vi "SaveHands_modified.vi"(8 "Error In":errorcluster, 11 ".NET Refnum in":refnum<k24>) -> (0 "Error Out":errorcluster, 3 "Left Hand":T1={"Palm Normal"={"Pitch"=nan, "Yaw"=nan, "Roll"=nan, "Magnitude"=nan, "XYZ"=[nan, nan, nan]}, "Palm Position"={"Pitch"=nan, "Yaw"=nan, "Roll"=nan, "Magnitude"=nan, "XYZ"=[nan, nan, nan]}, "Palm Velocity"={"Pitch"=nan, "Yaw"=nan, "Roll"=nan, "Magnitude"=nan, "XYZ"=[nan, nan, nan]}, "Direction"={"Pitch"=nan, "Yaw"=nan, "Roll"=nan, "Magnitude"=nan, "XYZ"=[nan, nan, nan]}, "Palm Position (Stabilized)"={"Pitch"=nan, "Yaw"=nan, "Roll"=nan, "Magnitude"=nan, "XYZ"=[nan, nan, nan]}, "Sphere Center"={"Pitch"=nan, "Yaw"=nan, "Roll"=nan, "Magnitude"=nan, "XYZ"=[nan, nan, nan]}, "Pointables"=[], "ID"=0, "Time Visible"=0.0, "Sphere Radius"=0.0})   [LabVIEW 2015]
uses:
  <vilib>/MakerHub/Leap/Private/Type Defs/Hand.ctl
  <vilib>/MakerHub/Leap/Private/Type Defs/Vector.ctl
  <vilib>/MakerHub/Leap/Private/Type Defs/Pointable.ctl
  <vilib>/MakerHub/Leap/Private/Type Defs/Pointable Type.ctl
  <vilib>/MakerHub/Leap/Private/Type Defs/Pointable Zone.ctl
  C:/Program Files (x86)/National Instruments/LabVIEW 2015/vi.lib/MakerHub/Leap/Private/Libs/LeapCSharp.NET3.5.dll
  Program Files (x86)/National Instruments/LabVIEW 2015/vi.lib/MakerHub/Leap/Private/Libs/LeapCSharp.NET3.5.dll
  <vilib>/MakerHub/Leap/LMH-Leap.lvlib
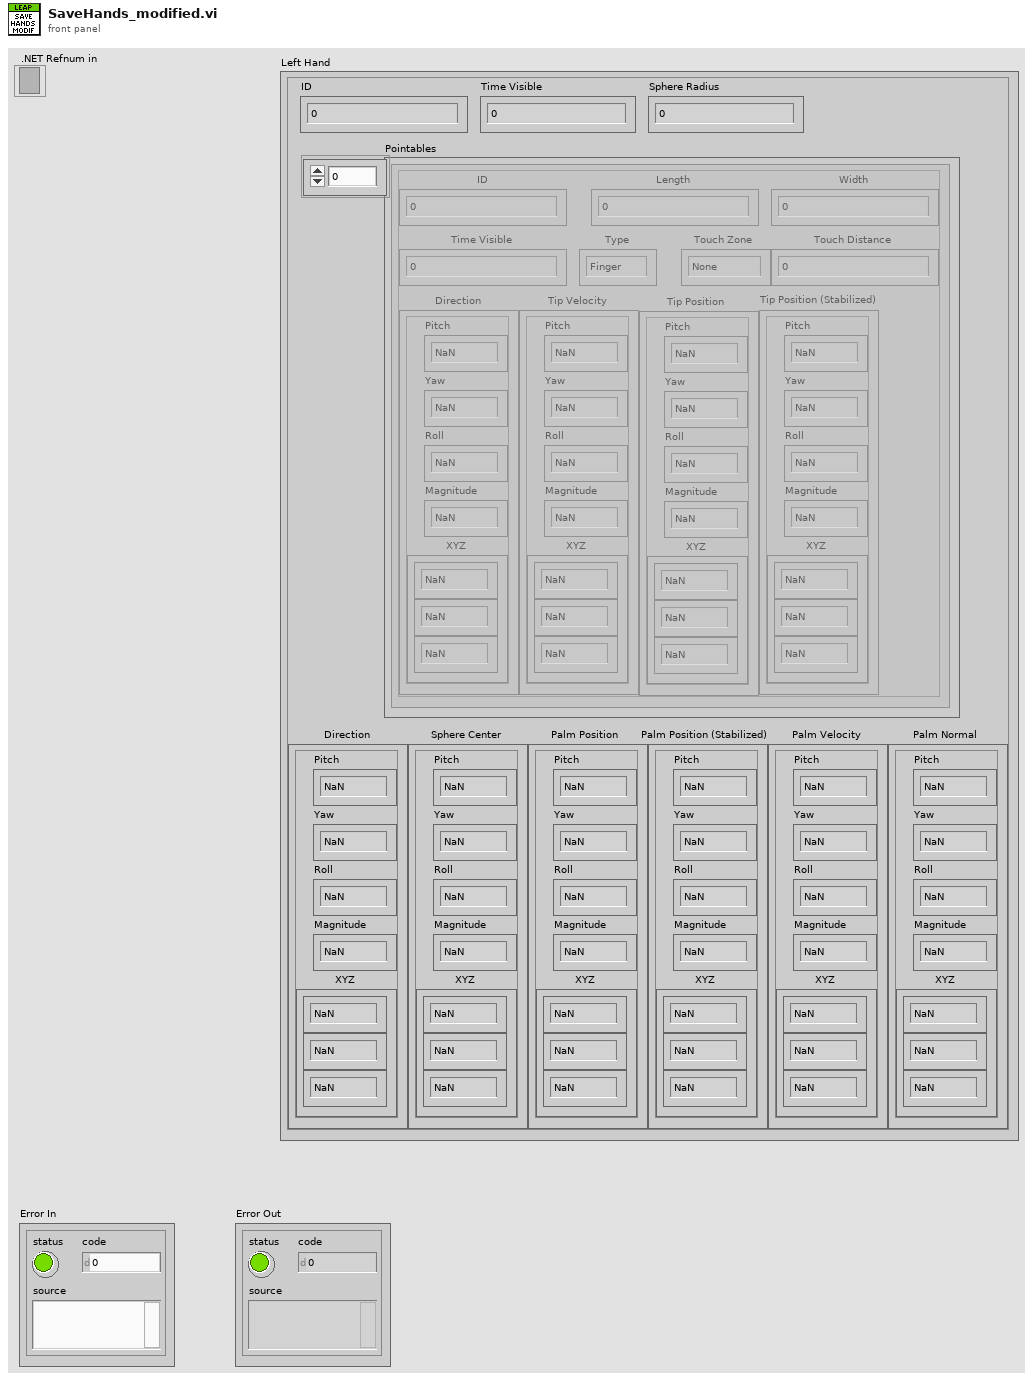
[diagram p1: front panel]
types:
  T1 = typedef "LMH-Leap.lvlib/Hand.ctl" = cluster{"Palm Normal":T2, "Palm Position":T2, "Palm Velocity":T2, "Direction":T2, "Palm Position (Stabilized)":T2, "Sphere Center":T2, "Pointables":T3[], "ID":i32, "Time Visible":sgl, "Sphere Radius":sgl}
  T2 = typedef "LMH-Leap.lvlib/Vector.ctl" = cluster{"Pitch":sgl, "Yaw":sgl, "Roll":sgl, "Magnitude":sgl, "XYZ":sgl[]}
  T3 = typedef "LMH-Leap.lvlib/Pointable.ctl" = cluster{"Type":T4, "Touch Zone":T5, "ID":i32, "Length":dbl, "Width":dbl, "Time Visible":dbl, "Touch Distance":dbl, "Direction":T2, "Tip Position":T2, "Tip Velocity":T2, "Tip Position (Stabilized)":T2}
  T4 = typedef "LMH-Leap.lvlib/Pointable Type.ctl" = enum16{"Finger", "Tool"}
  T5 = typedef "LMH-Leap.lvlib/Pointable Zone.ctl" = enum16{"None", "Hovering", "Touching"}
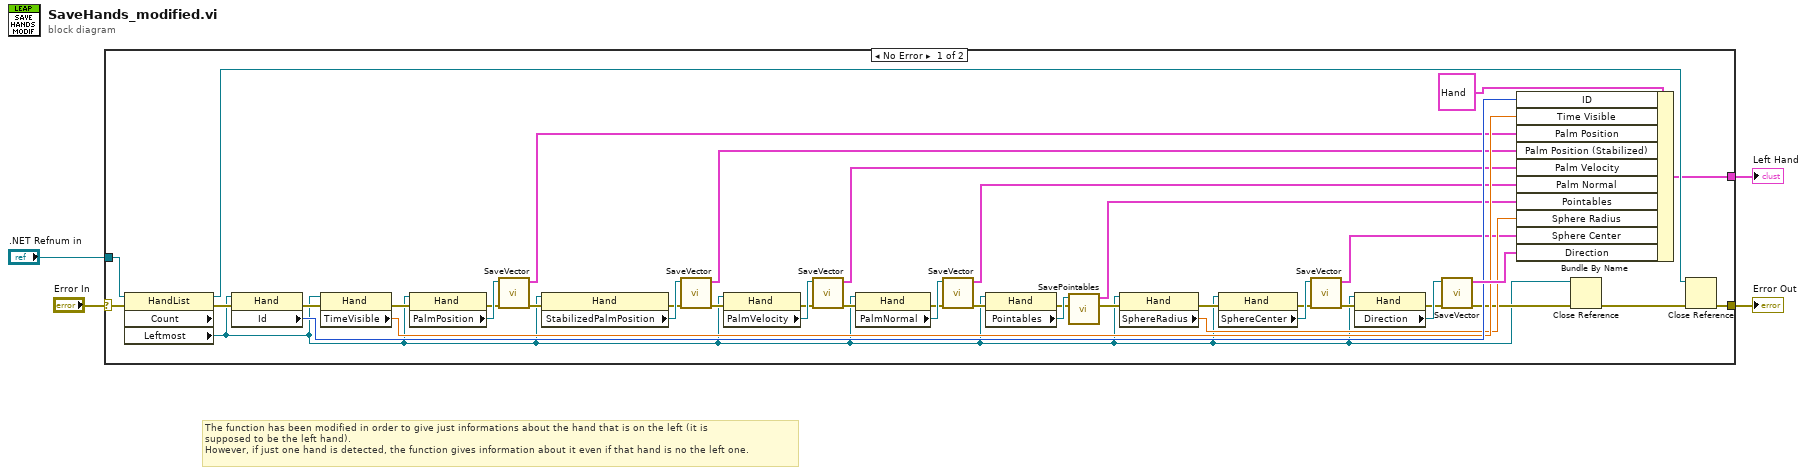
[diagram p0: block diagram]
diagram:
  # "The function has been modified in order to give just informations about the hand that is on the left (it is\nsupposed to be the left hand).\nHowever, if just one hand is detected, the function gives information about it even if that hand is no the left one."
  n1 = case shown="No Error" "Error In" {
    selector: "Error In" -> [w46 w48]
    tunnel: ".NET Refnum in" -> [w5 _]
    tunnel: [w44 w48] -> w3
    tunnel: [w8 _] -> w1
    frame No Error {
      n2 = property class="HandList" props=["Count", "Leftmost"](reference=w5, error in=w46) -> (reference out=w47:refnum<k24>, error out=w9:errorcluster, "Leftmost"=w6:refnum<k24>)  [unwired: 1 out]
      n3 = property class="Hand"(reference=w6, error in=w9) -> (error out=w41:errorcluster, "Id"=w38:i32)  [unwired: 1 out]
      n4 = property class="Hand"(reference=w6, error in=w41) -> (error out=w39:errorcluster, "TimeVisible"=w34:sgl)  [unwired: 1 out]
      n5 = property class="Hand"(reference=w6, error in=w39) -> (error out=w11:errorcluster, "PalmPosition"=w33:refnum<k24>)  [unwired: 1 out]
      n6 = call <vilib>:"SaveVector.vi"("error in (no error)"=w11, "Leap Vector"=w33) -> ("error out"=w10:errorcluster, "Vector"=w31:T2)  [unwired: 8 in]
      n7 = property class="Hand"(reference=w6, error in=w10) -> (error out=w12:errorcluster, "StabilizedPalmPosition"=w32:refnum<k24>)  [unwired: 1 out]
      n8 = call <vilib>:"SaveVector.vi"("error in (no error)"=w12, "Leap Vector"=w32) -> ("error out"=w13:errorcluster, "Vector"=w30:T2)  [unwired: 8 in]
      n9 = property class="Hand"(reference=w6, error in=w13) -> (error out=w14:errorcluster, "PalmVelocity"=w37:refnum<k24>)  [unwired: 1 out]
      n10 = call <vilib>:"SaveVector.vi"("error in (no error)"=w14, "Leap Vector"=w37) -> ("error out"=w15:errorcluster, "Vector"=w29:T2)  [unwired: 8 in]
      n11 = property class="Hand"(reference=w6, error in=w15) -> (error out=w16:errorcluster, "PalmNormal"=w36:refnum<k24>)  [unwired: 1 out]
      n12 = call <vilib>:"SaveVector.vi"("error in (no error)"=w16, "Leap Vector"=w36) -> ("error out"=w17:errorcluster, "Vector"=w28:T2)  [unwired: 8 in]
      n13 = property class="Hand"(reference=w6, error in=w17) -> (error out=w26:errorcluster, "Pointables"=w27:refnum<k24>)  [unwired: 1 out]
      n14 = call <vilib>:"SavePointables.vi"("error in (no error)"=w26, "Leap Pointables"=w27) -> ("error out"=w40:errorcluster, "Pointables"=w18:T3[])  [unwired: 8 in]
      n15 = property class="Hand"(reference=w6, error in=w40) -> (error out=w42:errorcluster, "SphereRadius"=w25:sgl)  [unwired: 1 out]
      n16 = property class="Hand"(reference=w6, error in=w42) -> (error out=w19:errorcluster, "SphereCenter"=w35:refnum<k24>)  [unwired: 1 out]
      n17 = call <vilib>:"SaveVector.vi"("error in (no error)"=w19, "Leap Vector"=w35) -> ("error out"=w20:errorcluster, "Vector"=w24:T2)  [unwired: 8 in]
      n18 = property class="Hand"(reference=w6, error in=w20) -> (error out=w21:errorcluster, "Direction"=w23:refnum<k24>)  [unwired: 1 out]
      n19 = call <vilib>:"SaveVector.vi"("error in (no error)"=w21, "Leap Vector"=w23) -> ("error out"=w22:errorcluster, "Vector"=w43:T2)  [unwired: 8 in]
      n20 = Bundle By Name(cluster=T1 {"Palm Normal"={"Pitch"=0.0, "Yaw"=0.0, "Roll"=0.0, "Magnitude"=0.0, "XYZ"=[]}, "Palm Position"={"Pitch"=0.0, "Yaw"=0.0, "Roll"=0.0, "Magnitude"=0.0, "XYZ"=[]}, "Palm Velocity"={"Pitch"=0.0, "Yaw"=0.0, "Roll"=0.0, "Magnitude"=0.0, "XYZ"=[]}, "Direction"={"Pitch"=0.0, "Yaw"=0.0, "Roll"=0.0, "Magnitude"=0.0, "XYZ"=[]}, "Palm Position (Stabilized)"={"Pitch"=0.0, "Yaw"=0.0, "Roll"=0.0, "Magnitude"=0.0, "XYZ"=[]}, "Sphere Center"={"Pitch"=0.0, "Yaw"=0.0, "Roll"=0.0, "Magnitude"=0.0, "XYZ"=[]}, "Pointables"=[], "ID"=0, "Time Visible"=0.0, "Sphere Radius"=0.0} ("Hand"), "ID"=w38, "Time Visible"=w34, "Palm Position"=w31, "Palm Position (Stabilized)"=w30, "Palm Velocity"=w29, "Palm Normal"=w28, "Pointables"=w18, "Sphere Radius"=w25, "Sphere Center"=w24, "Direction"=w43) -> (w8:T1)
      n21 = Close Reference(reference=w6, error in (no error)=w22) -> (error out=w45:errorcluster)
      n22 = Close Reference(reference=w47, error in (no error)=w45) -> (error out=w44:errorcluster)
    }
    frame Error {
    }
  }
  "Left Hand" <- w1
  "Error Out" <- w3
